vi "Compute Discrete Calibration Phasor & jw.vi"(8 "Laser Period (T)":dbl[unit], 9 "Calibration Lifetime (tau)":dbl[unit], 10 "# Gates (N)":dbl, 11 "Harmonic frequency (f)":dbl[unit]) -> (2 "Z_N(tau)":cdb, 3 "i 2 pi f (GHz)":cdb)   [LabVIEW 2019]
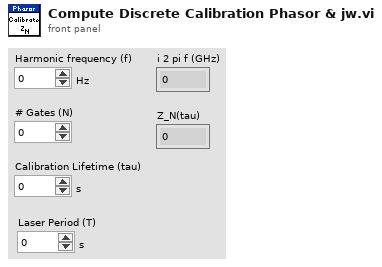
[diagram p1: front panel]
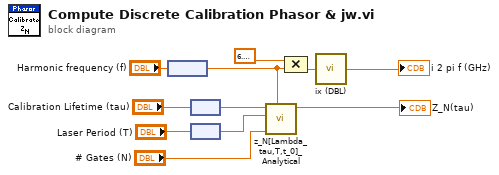
[diagram p0: block diagram]
diagram:
  n1 = node("Harmonic frequency (f)") -> (w5:dbl)
  n2 = node("Calibration Lifetime (tau)") -> (w6:dbl)
  n3 = node("Laser Period (T)") -> (w2:dbl)
  n4 = call "z_N[Lambda_tau,T,t_0]_Analytical.vi"("Harmonic f"=w5, "N"="# Gates (N)", "T"=w2, "tau"=w6) -> ("z"=→"Z_N(tau)":cxt)  [unwired: 7 in]
  n5 = Compound Arithmetic op=MULTIPLY(6.283185307179586, w5) -> (w11:dbl)
  n6 = call "ix (DBL).vi"("x (1)"=w11) -> ("ix"=→"i 2 pi f (GHz)":cdb)
